vi "ActionVIOnDelete.vi"(8 "error in (no error)":errorcluster, 10 "All deleted Refs":T1[](array[typedef]) format="%.0x", 11 "Item Ref in":T1 format="%.0x") -> (0 "error out":errorcluster, 3 "Item Ref out":T1 format="%.0x")   [LabVIEW 2020, in "SLSC EDS System Explorer.lvlib"]
uses:
  SLSC EDS System Explorer.lvlib
  <vilib>/NI VeriStand/Custom Device API/Custom Device Item Ref.ctl
  <vilib>/NI VeriStand/Custom Device API/Custom Device API.lvlib
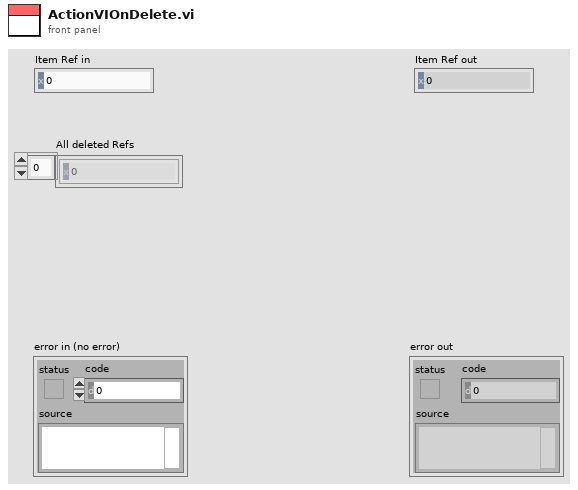
[diagram p1: front panel]
types:
  T1 = typedef "Custom Device API.lvlib/Custom Device Item Ref.ctl" = u64
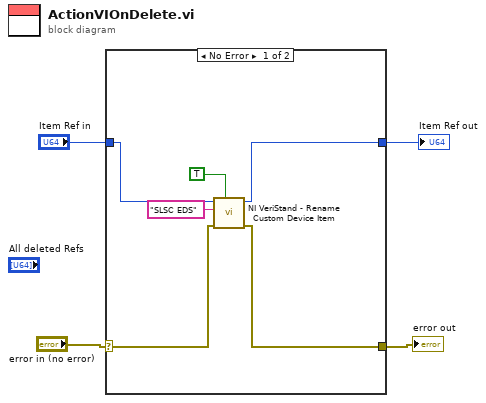
[diagram p0: block diagram]
diagram:
  n1 = case shown="No Error" "error in (no error)" {
    selector: "error in (no error)" -> [w7 w11]
    tunnel: [w8 w11] -> w3
    tunnel: [w9 w12] -> w2
    tunnel: "Item Ref in" -> [w10 w12]
    frame No Error {
      n2 = call <vilib>:"NI VeriStand - Rename Custom Device Item.vi"("Force Rename (F)"=TRUE, "error in (no error)"=w7, "New Name"="SLSC EDS", "Item Ref in"=w10) -> ("error out"=w8:errorcluster, "Item Ref out"=w9:T1)  [unwired: 6 out]
    }
    frame Error {
    }
  }
  "error out" <- w3
  "Item Ref out" <- w2
